vi "GV_FindAllAnalogs.vi"(9 "Bool_id in":bool[](array[boolean]), 11 "TAGproperties":T1=[{"TAG"="ch0001", "Qtype"="PAQ", "TAGprop"={"Description"="", "EngUnits"="", "RangeH"=-1.0, "RangeL"=-1.0, "Resolution"=-1, "Obsolete"=FALSE, "ChangeDate"=timestamp(3692433115.085 s since 1904-01-01), "ChangeSource"="AVPP", "ChangeReason"="100 Unidentified TAGs sent by HISW", "TagFunc"=0}}, {"TAG"="ch0002", "Qtype"="PAQ", "TAGprop"={"Description"="", "EngUnits"="", "RangeH"=-1.0, "RangeL"=-1.0, "Resolution"=-1, "Obsolete"=FALSE, "ChangeDate"=timestamp(3692433115.085 s since 1904-01-01), "ChangeSource"="AVPP", "ChangeReason"="100 Unidentified TAGs sent by HISW", "TagFunc"=0}}, {"TAG"="ch0003", "Qtype"="PAQ", "TAGprop"={"Description"="", "EngUnits"="", "RangeH"=-1.0, "RangeL"=-1.0, "Resolution"=-1, "Obsolete"=FALSE, "ChangeDate"=timestamp(3692433115.085 s since 1904-01-01), "ChangeSource"="AVPP", "ChangeReason"="100 Unidentified TAGs sent by HISW", "TagFunc"=0}}, {"TAG"="ch0005", "Qtype"="PAQ", "TAGprop"={"Description"="", "EngUnits"="", "RangeH"=-1.0, "RangeL"=-1.0, "Resolution"=-1, "Obsolete"=FALSE, "ChangeDate"=timestamp(3692433115.085 s since 1904-01-01), "ChangeSource"="AVPP", "ChangeReason"="100 Unidentified TAGs sent by HISW", "TagFunc"=0}}, {"TAG"="ch0006", "Qtype"="PAQ", "TAGprop"={"Description"="", "EngUnits"="", "RangeH"=-1.0, "RangeL"=-1.0, "Resolution"=-1, "Obsolete"=FALSE, "ChangeDate"=timestamp(3692433115.085 s since 1904-01-01), "ChangeSource"="AVPP", "ChangeReason"="100 Unidentified TAGs sent by HISW", "TagFunc"=0}}] {"TAGprop"."TagFunc" format="%08x"; "TAGprop"."RangeL" format="%.2f"; "TAGprop"."RangeH" format="%.2f"}) -> (1 "TypeIdxPerAnalogTag":i32[](array[numeric]), 2 "IndexPerType":cluster{"EngUnit":string, "IdxPerType":i32[]}[](array[cluster]), 3 "EngUnitTypes":string[](array[string]))   [LabVIEW 2020, in "Sgraph_lib_V1.lvlib" / "Gviewer.lvclass"]
doc: "Andre Koelewijn, 29 July 2022\n\nSearch for analog traces. Using this vi the code in this diagram can be formed like the identical autozoom part that is used to combine traces with identical engineering units.\nBy combining these parts the subsequent code remains identical."
uses:
  Gviewer.lvclass
  DBAL/controls/DBAL_TAGprops.ctl
  DBAL/controls/DBAL_TAGpropEdit.ctl
  Common/controls/typedef_com_TagProp.ctl
  Builds/Sgraph_lib_V1.lvlib
  DBAL/DBAL.lvclass
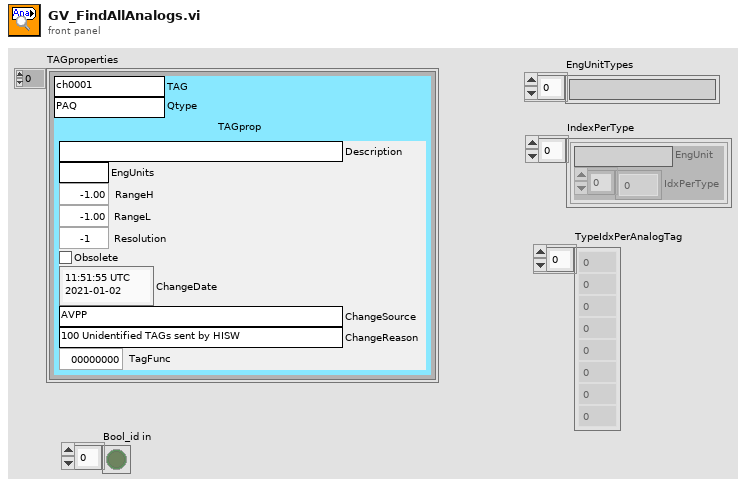
[diagram p1: front panel]
types:
  T1 = typedef "Sgraph_lib_V1.lvlib/DBAL.lvclass/DBAL_TAGprops.ctl" = T2[]
  T2 = typedef "Sgraph_lib_V1.lvlib/DBAL.lvclass/DBAL_TAGpropEdit.ctl" = cluster{"TAG":string, "Qtype":string, "TAGprop":T3}
  T3 = typedef "Sgraph_lib_V1.lvlib/typedef_com_TagProp.ctl" = cluster{"Description":string, "EngUnits":string, "RangeH":dbl, "RangeL":dbl, "Resolution":i32, "Obsolete":bool, "ChangeDate":timestamp, "ChangeSource":string, "ChangeReason":string, "TagFunc":u32}
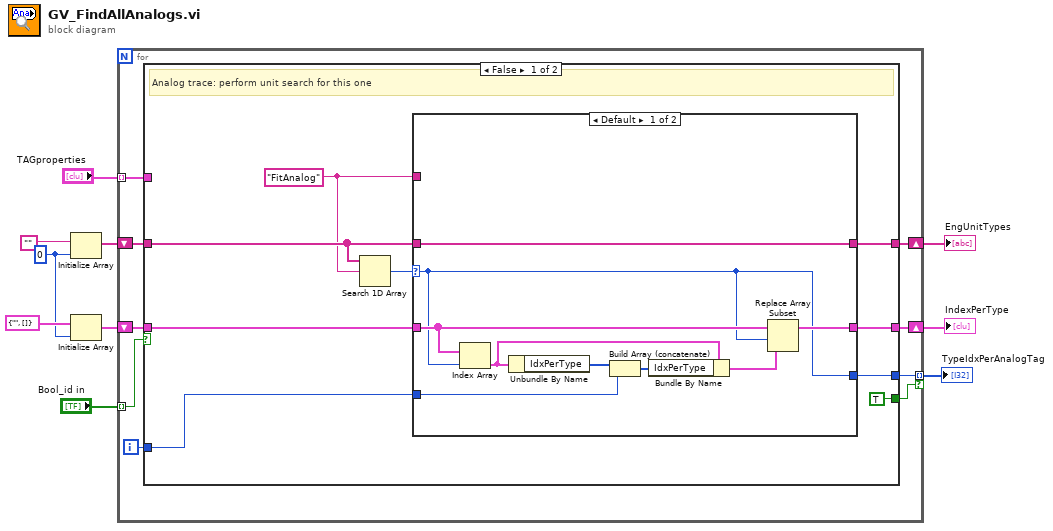
[diagram p0: block diagram]
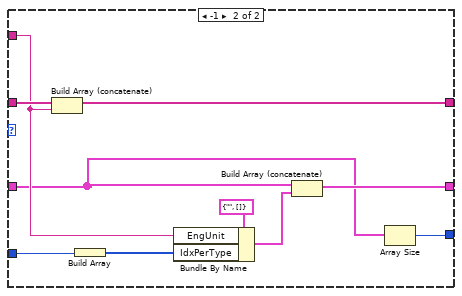
[diagram p2: hidden frame]
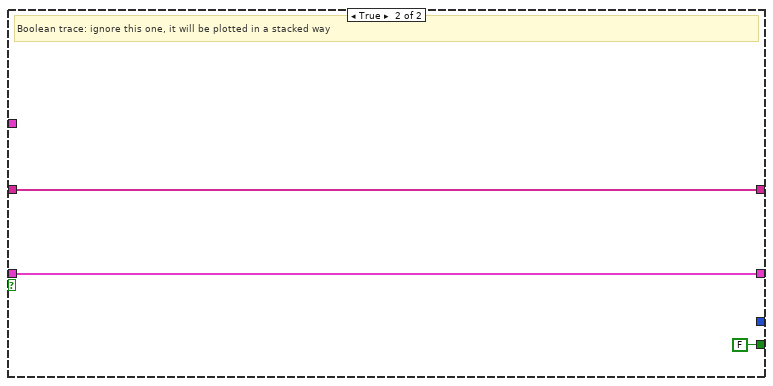
[diagram p3: hidden frame]
diagram:
  w5 = 0 ("dimension size")
  n1 = Initialize Array("", w5) -> (w8:string[])
  n2 = Initialize Array(cluster{"EngUnit":string, "IdxPerType":i32[]} {"EngUnit"="", "IdxPerType"=[]} ("IdxForOneType"), w5) -> (w4:cluster{"EngUnit":string, "IdxPerType":i32[]}[])
  n3 = for {
    tunnel: "TAGproperties" -> [w19] mode=indexing
    shift-right: [w17] -> w7
    shift-left: w8 -> [w18]
    shift-right: [w14] -> w3
    shift-left: w4 -> [w16]
    tunnel: [w13] -> w2 mode=indexing if=w11
    tunnel: "Bool_id in" -> [w12] mode=indexing
    i -> [w15]
    n4 = case shown="False" w12 {
      tunnel: w19 -> [_ _]
      tunnel: w18 -> [w27 w49]
      tunnel: [w26 w49] -> w17
      tunnel: w16 -> [w25 w50]
      tunnel: w15 -> [w24 _]
      tunnel: [w23 w50] -> w14
      tunnel: [w22 _] -> w13
      tunnel: [TRUE FALSE] -> w11
      frame False {
        w20 = "FitAnalog" ("string")
        # "Analog trace: perform unit search for this one"
        n5 = Search 1D Array(1D array=w27, element=w20) -> (index of element=w28:i32)  [unwired: 1 in]
        n6 = case shown="Default" w28 {
          selector: w28 -> [w29 _]
          tunnel: w20 -> [_ w43]
          tunnel: w27 -> [w37 w47]
          tunnel: [w37 w46] -> w26
          tunnel: w25 -> [w33 w39]
          tunnel: w24 -> [w30 w42]
          tunnel: [w31 w40] -> w23
          tunnel: [w29 w38] -> w22
          frame Default {
            n7 = Index Array(array=w33, index=w29) -> (element=w35:cluster{"EngUnit":string, "IdxPerType":i32[]})
            n8 = Unbundle By Name(w35) -> ("IdxPerType"=w36:i32[])
            n9 = Build Array (concatenate)(w36, w30) -> (w34:i32[])
            n10 = Bundle By Name(cluster=w35, "IdxPerType"=w34) -> (w32:cluster{"EngUnit":string, "IdxPerType":i32[]})
            n11 = Replace Array Subset(array=w33, new element=w32, index=w29) -> (w31:cluster{"EngUnit":string, "IdxPerType":i32[]}[])
          }
          frame -1 {
            n12 = Build Array (concatenate)(w47, w43) -> (w46:string[])
            n13 = Build Array(w42) -> (w41:i32[])
            n14 = Bundle By Name(cluster=cluster{"EngUnit":string, "IdxPerType":i32[]} {"EngUnit"="", "IdxPerType"=[]} ("IdxForOneType"), "EngUnit"=w43, "IdxPerType"=w41) -> (w44:cluster{"EngUnit":string, "IdxPerType":i32[]})
            n15 = Build Array (concatenate)(w39, w44) -> (w40:cluster{"EngUnit":string, "IdxPerType":i32[]}[])
            n16 = Array Size(array=w39) -> (size(s)=w38:i32)
          }
        }
      }
      frame True {
        # "Boolean trace: ignore this one, it will be plotted in a stacked way"
      }
    }
  }
  "IndexPerType" <- w3
  "EngUnitTypes" <- w7
  "TypeIdxPerAnalogTag" <- w2
